vi "国弘探头校准.vi"(3 "校准点位":u16(ring) caption="校准方式：" items=["第一点校准", "第二点校准", "第三点校准"], 5 "校准方式":u16, 6 "MB_Master输入":refnum<class "MB_Master.lvclass">, 7 "探头":T1(ring)=enum."氯化物", 8 "错误输入（无错误）":errorcluster, 9 "标液三":cluster{"标准值":dbl, "检测值":dbl, "原始值":dbl}, 10 "标液二":cluster{"标准值":dbl, "检测值":dbl, "原始值":dbl}, 11 "标液一":cluster{"标准值":dbl, "检测值":dbl, "原始值":dbl}) -> (0 "错误输出":errorcluster)   [LabVIEW 2016, in "斯坦道多参数.lvlib"]
uses:
  <vilib>/Plasmionique/MB Master/MB_Master/MB_Master.lvclass
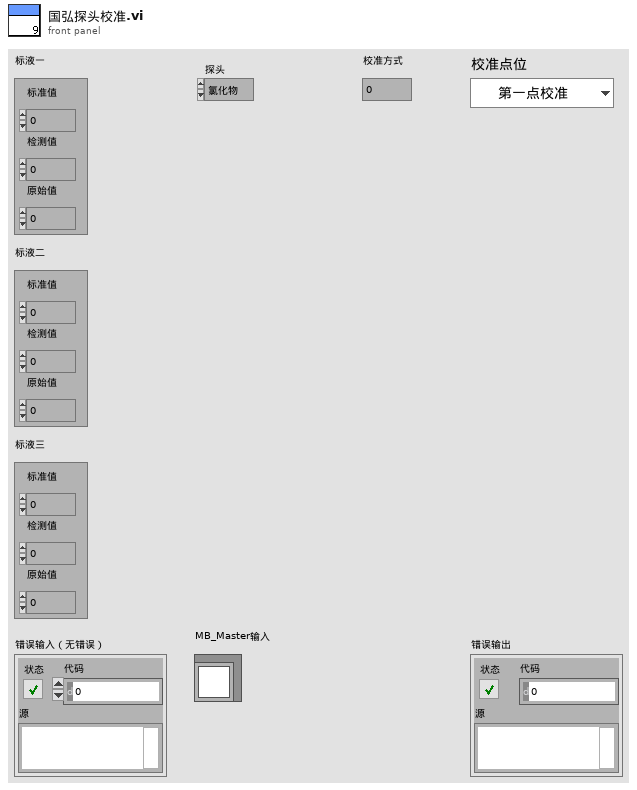
[diagram p1: front panel]
types:
  T1 = enum16{"NULL", "pH", "Cond", "DO", "Turb", "ORP", "6", "7", "COD", "9", "氯化物", "11", "12", "13", "14", "15", "16", "水中油"}
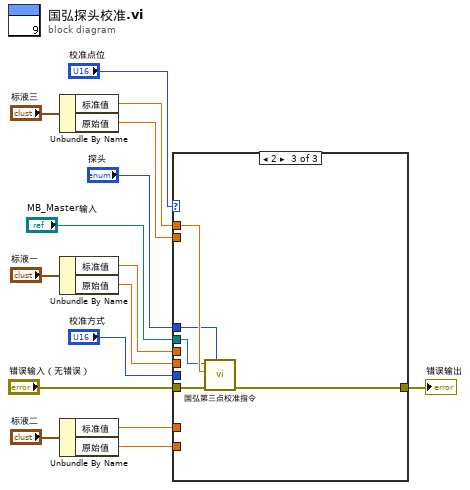
[diagram p0: block diagram]
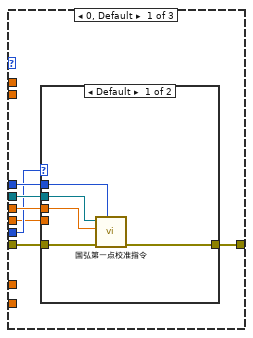
[diagram p2: hidden frame]
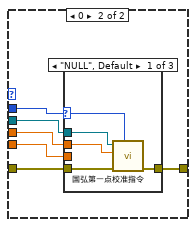
[diagram p3: hidden frame]
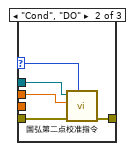
[diagram p4: hidden frame]
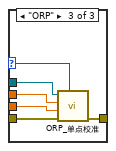
[diagram p5: hidden frame]
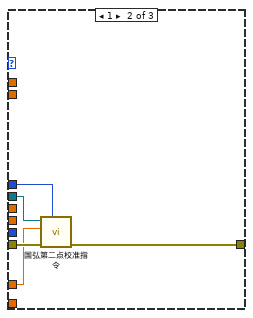
[diagram p6: hidden frame]
diagram:
  n1 = Unbundle By Name("标液三") -> ("标准值"=w14:dbl, "原始值"=w15:dbl)
  n2 = Unbundle By Name("标液一") -> ("标准值"=w10:dbl, "原始值"=w11:dbl)
  n3 = Unbundle By Name("标液二") -> ("标准值"=w12:dbl, "原始值"=w13:dbl)
  n4 = case shown="2" "校准点位" {
    tunnel: "MB_Master输入" -> [w22 w51 w57]
    tunnel: "错误输入（无错误）" -> [w20 w54 w59]
    tunnel: w10 -> [w21 _ _]
    tunnel: w11 -> [w16 _ _]
    tunnel: w12 -> [_ w50 _]
    tunnel: w13 -> [_ _ _]
    tunnel: w14 -> [_ _ w58]
    tunnel: w15 -> [_ _ _]
    tunnel: [w19 w53 w56] -> w4
    tunnel: "探头" -> [w18 w52 w55]
    tunnel: "校准方式" -> [w17 _ _]
    frame 0, Default {
      n5 = case shown="Default" w17 {
        tunnel: w22 -> [w24 w33]
        tunnel: w21 -> [w25 w32]
        tunnel: w20 -> [w27 w31]
        tunnel: [w26 w30] -> w19
        tunnel: w18 -> [w23 w29]
        tunnel: w16 -> [_ w28]
        frame Default {
          n6 = call "国弘第一点校准指令.vi"("探头"=w23, "error in (no error)"=w27, "标准值"=w25, "MB session in"=w24) -> ("error out"=w26:errorcluster)  [unwired: 6 in, 1 out]
        }
        frame 0 {
          n7 = case shown="\"NULL\", Default" w29 {
            selector: w29 -> [w34 w40 w46]
            tunnel: w33 -> [w38 w43 w49]
            tunnel: w32 -> [w37 w41 w48]
            tunnel: w31 -> [w36 w42 w44]
            tunnel: [w35 w39 w45] -> w30
            tunnel: w28 -> [_ _ w47]
            frame "NULL", Default {
              n8 = call "国弘第一点校准指令.vi"("探头"=w34, "error in (no error)"=w36, "标准值"=w37, "MB session in"=w38) -> ("error out"=w35:errorcluster)  [unwired: 6 in, 1 out]
            }
            frame "Cond", "DO" {
              n9 = call "国弘第二点校准指令.vi"("探头"=w40, "error in (no error)"=w42, "标准值"=w41, "MB session in"=w43) -> ("error out"=w39:errorcluster)  [unwired: 6 in, 1 out]
            }
            frame "ORP" {
              n10 = call "ORP_单点校准.vi"("探头"=w46, "error in (no error)"=w44, "信号值"=w47, "标准值"=w48, "MB session in"=w49) -> ("error out"=w45:errorcluster)  [unwired: 5 in, 1 out]
            }
          }
        }
      }
    }
    frame 1 {
      n11 = call "国弘第二点校准指令.vi"("探头"=w52, "error in (no error)"=w54, "标准值"=w50, "MB session in"=w51) -> ("error out"=w53:errorcluster)  [unwired: 6 in, 1 out]
    }
    frame 2 {
      n12 = call "国弘第三点校准指令.vi"("探头"=w55, "error in (no error)"=w59, "标准值"=w58, "MB session in"=w57) -> ("error out"=w56:errorcluster)  [unwired: 6 in, 1 out]
    }
  }
  "错误输出" <- w4
